vi "read test info.vi"(8 "错误输入（无错误）":errorcluster, 11 "tdms file in":refnum<k34>) -> (0 "错误输出":errorcluster, 1 "测试条件":T2, 2 "粉尘特性":T1, 3 "TDMS文件输出":refnum<k34>)   [LabVIEW 2011]
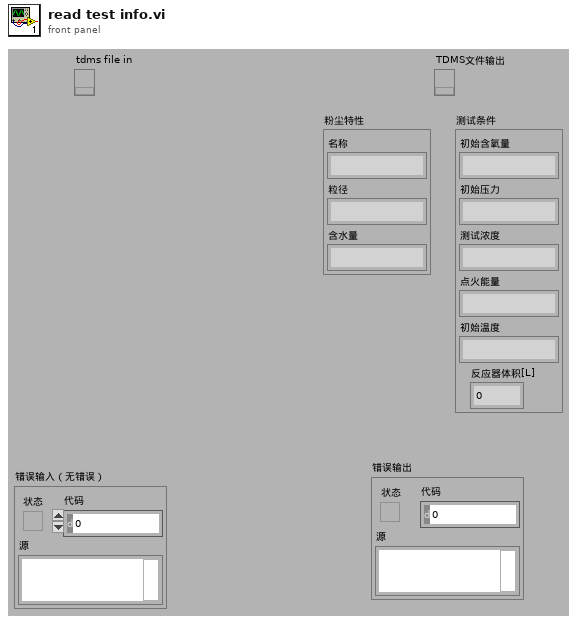
[diagram p1: front panel]
types:
  T1 = typedef "粉尘特性.ctl" = cluster{"名称":string, "粒径":string, "含水量":string}
  T2 = typedef "测试条件.ctl" = cluster{"初始含氧量":string, "初始压力":string, "测试浓度":string, "点火能量":string, "初始温度":string, "反应器体积[L]":dbl}
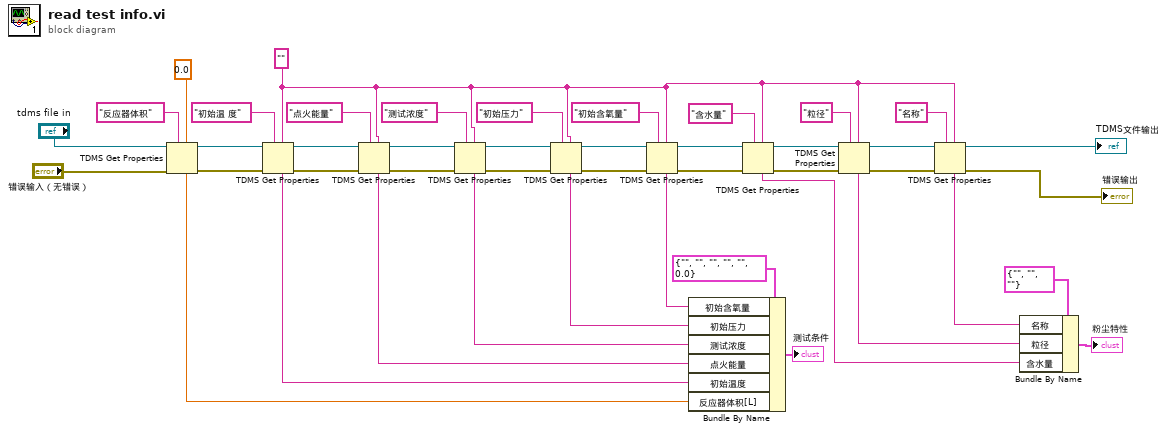
[diagram p0: block diagram]
diagram:
  w11 = "" ("数据类型")
  n1 = TDMS Get Properties(5:0.0 ("反应器体积[L]"), 7:"反应器体积", 8:"错误输入（无错误）", 11:"tdms file in") -> (0:w43:errorcluster, 3:w35:refnum<k34>, 4:w13:dbl)  [unwired: 5 out]
  n2 = TDMS Get Properties(5:w11, 7:"初始温 度", 8:w43, 11:w35) -> (0:w42:errorcluster, 3:w34:refnum<k34>, 4:w12:string)  [unwired: 5 out]
  n3 = TDMS Get Properties(5:w11, 7:"点火能量", 8:w42, 11:w34) -> (0:w41:errorcluster, 3:w33:refnum<k34>, 4:w6:string)  [unwired: 5 out]
  n4 = TDMS Get Properties(5:w11, 7:"测试浓度", 8:w41, 11:w33) -> (0:w40:errorcluster, 3:w32:refnum<k34>, 4:w7:string)  [unwired: 5 out]
  n5 = TDMS Get Properties(5:w11, 7:"初始压力", 8:w40, 11:w32) -> (0:w39:errorcluster, 3:w31:refnum<k34>, 4:w8:string)  [unwired: 5 out]
  n6 = TDMS Get Properties(5:w11, 7:"初始含氧量", 8:w39, 11:w31) -> (0:w38:errorcluster, 3:w30:refnum<k34>, 4:w9:string)  [unwired: 5 out]
  n7 = Bundle By Name(cluster=T2 {"初始含氧量"="", "初始压力"="", "测试浓度"="", "点火能量"="", "初始温度"="", "反应器体积[L]"=0.0} ("测试条件"), "初始含氧量"=w9, "初始压力"=w8, "测试浓度"=w7, "点火能量"=w6, "初始温度"=w12, "反应器体积[L]"=w13) -> (→"测试条件":T2)
  n8 = TDMS Get Properties(5:w11, 7:"含水量" ("属性名称"), 8:w38, 11:w30) -> (0:w37:errorcluster, 3:w29:refnum<k34>, 4:w2:string)  [unwired: 5 out]
  n9 = TDMS Get Properties(5:w11, 7:"粒径" ("属性名称"), 8:w37, 11:w29) -> (0:w36:errorcluster, 3:w28:refnum<k34>, 4:w3:string)  [unwired: 5 out]
  n10 = TDMS Get Properties(5:w11, 7:"名称" ("属性名称"), 8:w36, 11:w28) -> (0:→"错误输出":errorcluster, 3:→"TDMS文件输出":refnum<k34>, 4:w4:string)  [unwired: 5 out]
  n11 = Bundle By Name(cluster=T1 {"名称"="", "粒径"="", "含水量"=""} ("粉尘特性"), "名称"=w4, "粒径"=w3, "含水量"=w2) -> (→"粉尘特性":T1)
